vi "galvoRun.vi"() -> ()   [LabVIEW 2017]
panel:
  in  "write X (T)":bool=TRUE
  in  "write Y (T)":bool
  in  "stop":bool
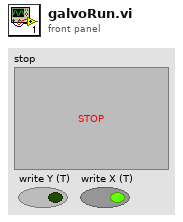
[diagram p1: front panel]
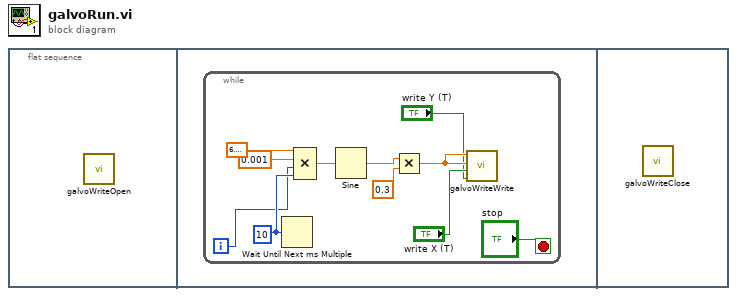
[diagram p0: block diagram]
diagram:
  n1 = flat-sequence {
    frame #0 {
      n2 = call "galvoWriteOpen.vi"() -> ()  [unwired: 12 in]
    }
    frame #1 {
      n3 = while {
        i -> [w8]
        stop <- "stop" stop-if-true
        w9 = u32 10 ("millisecond multiple")
        n4 = Wait Until Next ms Multiple(millisecond multiple=w9) -> ()  [unwired: 1 out]
        n5 = Compound Arithmetic op=MULTIPLY(6.283185307179586, 0.001 ("value"), w8, w9) -> (w6:dbl)
        n6 = Sine(x=w6) -> (sin(x)=w5:dbl)
        n7 = Multiply(x=w5, y=0.3) -> (x*y=w2:dbl)
        n8 = call "galvoWriteWrite.vi"("X"=w2, "Y"=w2, "write X (T)"="write X (T)", "write Y (T)"="write Y (T)") -> ()  [unwired: 2 in]
      }
    }
    frame #2 {
      n9 = call "galvoWriteClose.vi"() -> ()  [unwired: 12 in]
    }
  }
